vi "Tugas Function HUI.vi"() -> ()   [LabVIEW 2021]
uses:
  <vilib>/addons/Control Design/_Model Construction/Data Typedefs.llb/CD Time Info.ctl
  <vilib>/addons/Control Design/_Model Construction/Model Creation.llb/Model Creation SubVI/cd_Create Transfer Function Model.vi
  <vilib>/addons/Control Design/_Model Interconnection/Model Interconnection.llb/Model Interconnection SubVI/cd_Unit Feedback (TF and TF).vi
  <vilib>/addons/Control Design/_Model Interconnection/Model Interconnection.llb/Model Interconnection SubVI/cd_Series (TF and TF).vi
  <vilib>/addons/Control Design/_Model Interconnection/Model Interconnection.llb/Model Interconnection SubVI/cd_Parallel (TF and TF).vi
  <vilib>/addons/Control Design/_Model Interconnection/Model Interconnection.llb/Model Interconnection SubVI/cd_Feedback (TF and TF).vi
  <vilib>/addons/Control Design/_Dynamic Analysis/Dynamic Analysis.llb/Dynamic Analysis subVI/cd_Pole-Zero Map (Transfer Function).vi
  <vilib>/addons/Control Design/_Utility/Model Viewer.llb/Model Viewer SubVI/cd_Draw Transfer Function Equation (TF).vi
  <vilib>/addons/Control Design/_Time Response Analysis/Time Response.llb/Time Response subVI/cd_Step Response (Transfer Function).vi
  <vilib>/addons/Control Design/_Model Construction/NI_LinSys_Model Creation.lvlib
  <vilib>/addons/Control Design/_Model Interconnection/NI_CD_Model Interconnection.lvlib
  <vilib>/addons/Control Design/_Utility/NI_CD_Model Viewer.lvlib
  <vilib>/addons/Control Design/_Time Response Analysis/NI_CD_Time Response.lvlib
  <vilib>/addons/Control Design/_Dynamic Analysis/NI_CD_Dynamic Analysis.lvlib
  <vilib>/addons/Control Design/_Model Construction/NI_LinSys_Data Typedefs.lvlib
panel:
  in  "Mapping Output":T1(tab)
  out "Equation":picture
  out "Step Response Graph":cluster{"time":dbl[], dbl[]}[](graph)
  out "Pole-Zero Map":cluster{dbl[], dbl[]}[](graph)
  out "Poles":cdb[](array[numeric]) format="%.4f"
  out "Zeros":cdb[](array[numeric]) format="%.4f"
  in  "Tab Control 3":enum32{"Control Panel", "Setting Function"}(tab)
  in  "Tab Control 2":enum32{"Page 1", "Page 2"}(tab)
  in  "Setting":bool
  in  "Username":string
  in  "Password":string
  in  "Type Calculate":T2(ring)
  in  "Exit":bool
  in  "Show Output":T3(ring)
  in  "Login":bool
  in  "Tab Control":enum32{"Page 1", "Page 2"}(tab)
  in  "Numerator of G(s)":dbl[](array[numeric]) format="%#.5g"
  in  "Denominator of G(s)":dbl[](array[numeric]) format="%#.5g"
  in  "Numerator of Gc(s)":dbl[](array[numeric]) format="%#.5g"
  in  "Denominator of Gc(s)":dbl[](array[numeric]) format="%#.5g"
  in  "Time Range":T4={"t0"=-1.0, "dt"=-1.0, "tf"=-1.0} {"dt" format="%#.6g"; "tf" format="%#.6g"; "t0" format="%#.6g"}
  in  "Back":bool
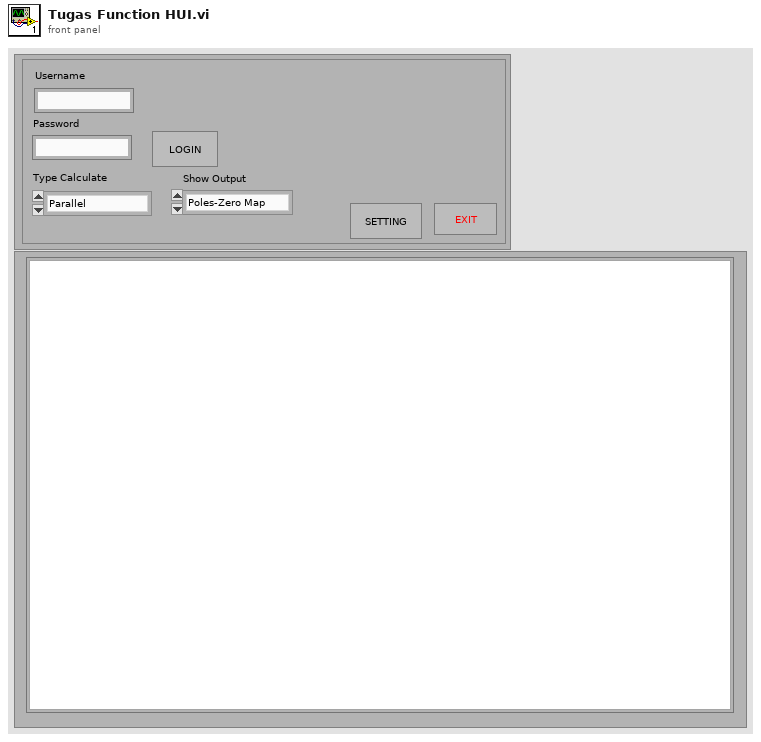
[diagram p1: front panel]
types:
  T1 = enum32{" Equation", "Step Function", "Poles-Zero Map"}
  T2 = enum16{"Parallel", "Series", "Feedback", "Unit Feedback"}
  T3 = enum16{"Poles-Zero Map", "Step Function", "Equation"}
  T4 = typedef "NI_LinSys_Data Typedefs.lvlib/CD Time Info.ctl" = cluster{"t0":dbl, "dt":dbl, "tf":dbl}
  T5 = typedef "NI_LinSys_Model Typedefs.lvlib/CD Transfer Function Model (MIMO).ctl" = cluster{"properties":T6, "transfer function(s)":T7[][]}
  T6 = typedef "NI_LinSys_Model Typedefs.lvlib/CD General Elements.ctl" = cluster{"Model name":string, "Input names":string[], "Output names":string[], "Input Delays":dbl[], "Output Delays":dbl[], "Sampling Time":dbl, "Notes":string}
  T7 = typedef "NI_LinSys_Model Typedefs.lvlib/CD Transfer Function Model (SISO).ctl" = cluster{"Numerator":dbl[], "Denominator":dbl[], "delay":dbl}
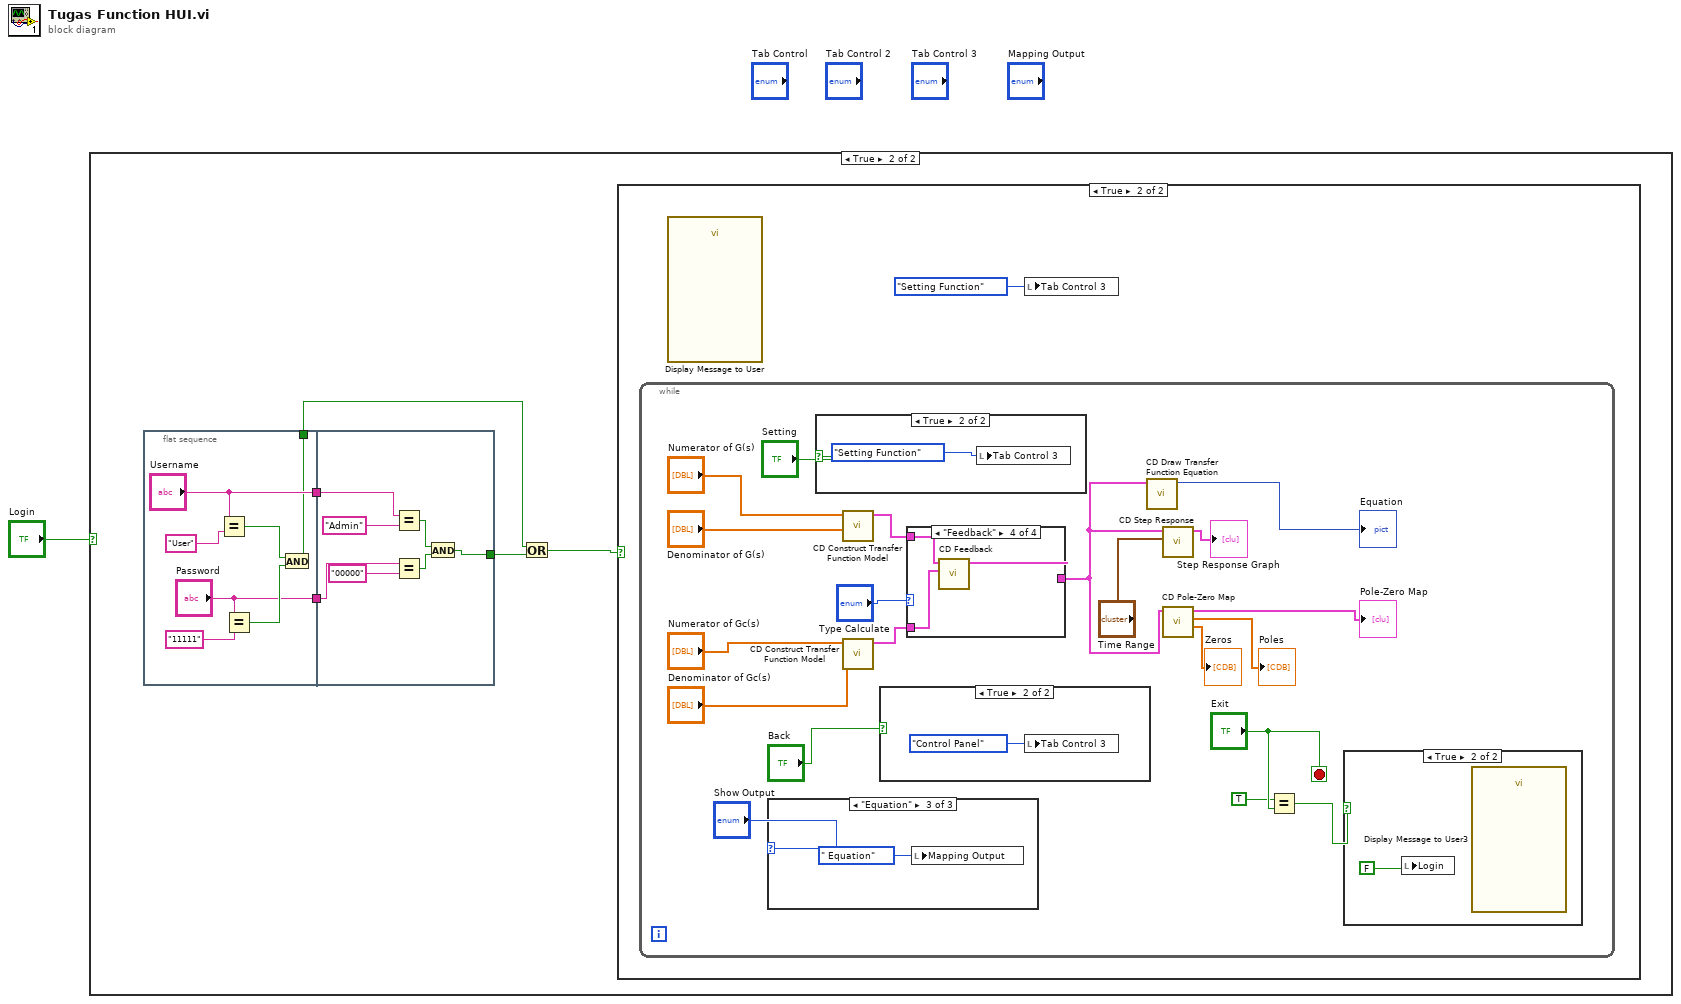
[diagram p0: block diagram]
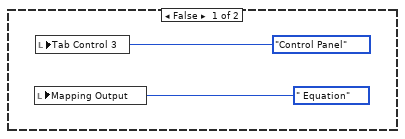
[diagram p2: hidden frame]
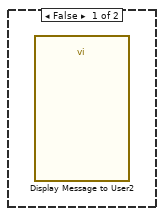
[diagram p3: hidden frame]
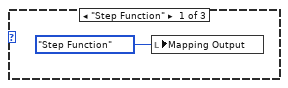
[diagram p6: hidden frame]
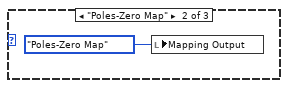
[diagram p7: hidden frame]
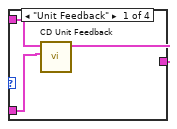
[diagram p9: hidden frame]
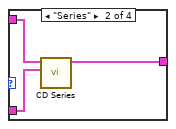
[diagram p10: hidden frame]
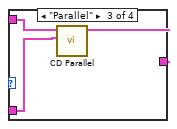
[diagram p11: hidden frame]
diagram:
  n1 = case shown="True" "Login" {
    frame False {
      n2 = local write "Mapping Output"(T1." Equation" ("Mapping Output")) -> ()
      n3 = local write "Tab Control 3"(enum32{"Control Panel", "Setting Function"}."Control Panel" ("Tab Control 3")) -> ()
    }
    frame True {
      n4 = flat-sequence {
        tunnel: ["Username"] -> w8
        tunnel: ["Password"] -> w7
        tunnel: [w48] -> w6
        tunnel: w8 -> [w59]
        tunnel: w7 -> [w58]
        tunnel: [w55] -> w5
        frame #0 {
          n5 = Equal?(x="Username", y="User") -> (x = y?=w52:bool)
          n6 = Equal?(x="Password", y="11111") -> (x = y?=w51:bool)
          n7 = And(x=w52, y=w51) -> (x .and. y?=w48:bool)
        }
        frame #1 {
          n8 = Equal?(x=w59, y="Admin") -> (x = y?=w61:bool)
          n9 = Equal?(x=w58, y="00000") -> (x = y?=w60:bool)
          n10 = And(x=w61, y=w60) -> (x .and. y?=w55:bool)
        }
      }
      n11 = Or(x=w6, y=w5) -> (x .or. y?=w4:bool)
      n12 = case shown="True" w4 {
        frame False {
          n13 = call "Display Message to User2"() -> ()  [unwired: 10 in, 2 out]
        }
        frame True {
          n14 = while {
            stop <- "Exit" stop-if-true
            n15 = case shown="\"Equation\"" "Show Output" {
              frame "Step Function" {
                n16 = local write "Mapping Output"(T1."Step Function" ("Mapping Output")) -> ()
              }
              frame "Poles-Zero Map" {
                n17 = local write "Mapping Output"(T1."Poles-Zero Map" ("Mapping Output")) -> ()
              }
              frame "Equation" {
                n18 = local write "Mapping Output"(T1." Equation" ("Mapping Output")) -> ()
              }
            }
            n19 = case shown="True" "Setting" {
              frame False {
              }
              frame True {
                n20 = local write "Tab Control 3"(enum32{"Control Panel", "Setting Function"}."Setting Function" ("Tab Control 3")) -> ()
              }
            }
            n21 = call-poly <vilib>:"CD Construct Transfer Function Model.vi"("Denominator"="Denominator of G(s)", "Numerator"="Numerator of G(s)") -> ("Transfer Function Model"=w25:T5)  [unwired: 8 in, 1 out]
            n22 = call-poly <vilib>:"CD Construct Transfer Function Model.vi"("Denominator"="Denominator of Gc(s)", "Numerator"="Numerator of Gc(s)") -> ("Transfer Function Model"=w24:T5)  [unwired: 8 in, 1 out]
            n23 = case shown="True" "Back" {
              frame False {
              }
              frame True {
                n24 = local write "Tab Control 3"(enum32{"Control Panel", "Setting Function"}."Control Panel" ("Tab Control 3")) -> ()
              }
            }
            n25 = case shown="\"Feedback\"" "Type Calculate" {
              tunnel: w25 -> [w38 w41 w44 w47]
              tunnel: w24 -> [w37 w40 w43 w46]
              tunnel: [w36 w39 w42 w45] -> w16
              frame "Unit Feedback" {
                n26 = call-poly <vilib>:"CD Unit Feedback.vi"("Model 2"=w37, "Model 1"=w38) -> ("Closed-Loop Model"=w36:T5)  [unwired: 8 in, 1 out]
              }
              frame "Series" {
                n27 = call-poly <vilib>:"CD Series.vi"("Model 2"=w40, "Model 1"=w41) -> ("Series Model"=w39:T5)  [unwired: 8 in, 1 out]
              }
              frame "Parallel" {
                n28 = call-poly <vilib>:"CD Parallel.vi"("Model 2"=w43, "Model 1"=w44) -> ("Parallel Model"=w42:T5)  [unwired: 8 in, 1 out]
              }
              frame "Feedback" {
                n29 = call-poly <vilib>:"CD Feedback.vi"("Model 2"=w46, "Model 1"=w47) -> ("Closed-Loop Model"=w45:T5)  [unwired: 8 in, 1 out]
              }
            }
            n30 = call-poly <vilib>:"CD Draw Transfer Function Equation.vi"("Transfer Function Model"=w16) -> ("Equation"=→"Equation":picture)  [unwired: 8 in, 2 out]
            n31 = call-poly <vilib>:"CD Step Response.vi"("Time Range"="Time Range", "Transfer Function Model"=w16) -> ("Step Response Graph"=→"Step Response Graph":cluster{"time":dbl[], dbl[]}[])  [unwired: 7 in, 2 out]
            n32 = call-poly <vilib>:"CD Pole-Zero Map.vi"("Transfer Function Model"=w16) -> ("Zeros"=→"Zeros":cdb[], "Poles"=→"Poles":cdb[], "Pole-Zero Map"=→"Pole-Zero Map":cluster{dbl[], dbl[]}[])  [unwired: 7 in, 1 out]
            n33 = Equal?(x=TRUE, y="Exit") -> (x = y?=w13:bool)
            n34 = case shown="True" w13 {
              frame False {
              }
              frame True {
                n35 = local write "Login"(FALSE) -> ()
                n36 = call "Display Message to User3"() -> ()  [unwired: 10 in, 2 out]
              }
            }
          }
          n37 = call "Display Message to User"() -> ()  [unwired: 10 in, 2 out]
          n38 = local write "Tab Control 3"(enum32{"Control Panel", "Setting Function"}."Setting Function" ("Tab Control 3")) -> ()
        }
      }
    }
  }
